vi "CoreCommand.vi"(0 "Serial Device in":refnum<class "Serial Device.lvclass">, 1 "Serial Device Brand":string, 5 "Command":string(combo), 7 "Param 1":string, 9 "Param 2":string, 11 "error in (no error)":errorcluster) -> (4 "Serial Device out":refnum<class "Serial Device.lvclass">, 6 "Command to send":string, 8 "Expected Command":string, 15 "error out":errorcluster)   [LabVIEW 2020, in "Serial Device.lvclass"]
uses:
  Serial Device.lvclass
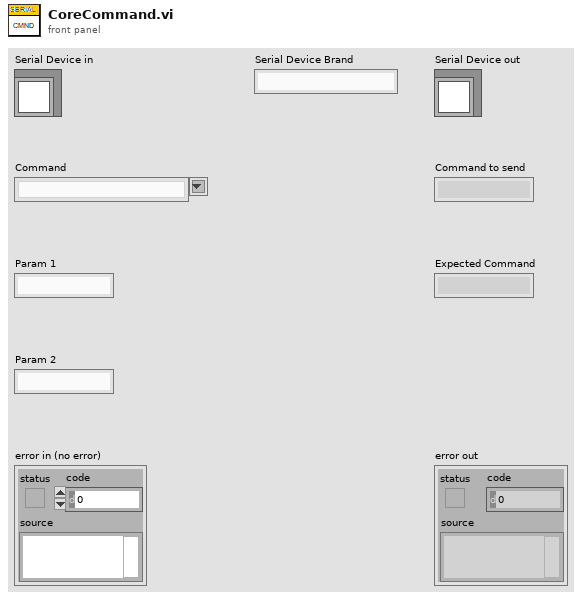
[diagram p1: front panel]
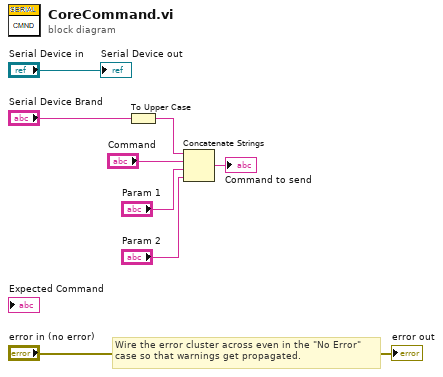
[diagram p0: block diagram]
diagram:
  # "Wire the error cluster across even in the \"No Error\"\ncase so that warnings get propagated."
  n1 = To Upper Case(1:"Serial Device Brand") -> (0:w5:string)
  n2 = Concatenate Strings(w5, "Command", "Param 1", "Param 2") -> (→"Command to send":string)
  "error out" <- "error in (no error)"
  "Serial Device out" <- "Serial Device in"
